vi "Format Log Data.vi"(11 "Array in":i16[](array[numeric])) -> (3 "Array out":i16[][](array[numeric]))   [LabVIEW 2017, in "HostCode.lvlib"]
uses:
  HostCode.lvlib
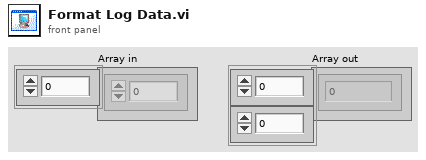
[diagram p1: front panel]
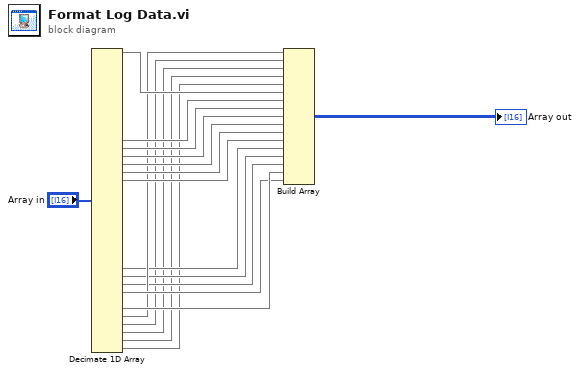
[diagram p0: block diagram]
diagram:
  n1 = Decimate 1D Array("Array in") -> (w17:i16[], w10:i16[], w11:i16[], w12:i16[], w13:i16[], w14:i16[], w18:i16[], w8:i16[], w7:i16[], w6:i16[], w15:i16[], w16:i16[], w9:i16[], w2:i16[], w3:i16[], w4:i16[], w5:i16[])  [unwired: 21 out]
  n2 = Build Array(w9, w2, w3, w4, w5, w17, w10, w11, w12, w13, w14, w18, w8, w7, w6, w16, w15) -> (→"Array out":i16[][])
